vi "Datum draw.vi"(8 "error in (no error)":errorcluster, 10 "Details in":T1={"Angle"=0.0, "Reference"="", "Xoffset"=0, "Arc size"=0.0, "Measurment Name"="", "Pixel density"=0.0, "Circle"={"Point 1"={"X"=0.0, "Y"=0.0}, "Point 2"={"X"=0.0, "Y"=0.0}, "Center (Pixels)"={"X"=0.0, "Y"=0.0}, "Radius (Pixels)"=0.0}, "Color"=0, "Slanting line start"={"X"=0.0, "Y"=0.0}, "Sleeping line start"={"X"=0.0, "Y"=0.0}, "Mouse release"={"X"=0.0, "Y"=0.0}, "Line width"=0, "Small FOV?"=FALSE, "Fixed overlay details"={"Overlay coordinates"=[], "Config coordinates"=[], "Inspection mode?"=TRUE}, "PM angle"=0.0}, 11 "Image in":T2) -> (0 "error out":errorcluster, 1 "Overlay coordinates out":cluster{"X":dbl, "Y":dbl}[](array[cluster]), 2 "Text origin":cluster{"X":sgl, "Y":sgl}, 3 "Image out":T2)   [LabVIEW 2019]
uses:
  <vilib>/vision/Image Controls.llb/IMAQ Image.ctl
  Controls/DatumLine draw.ctl
  <vilib>/vision/NI_Vision_Development_Module.lvlib
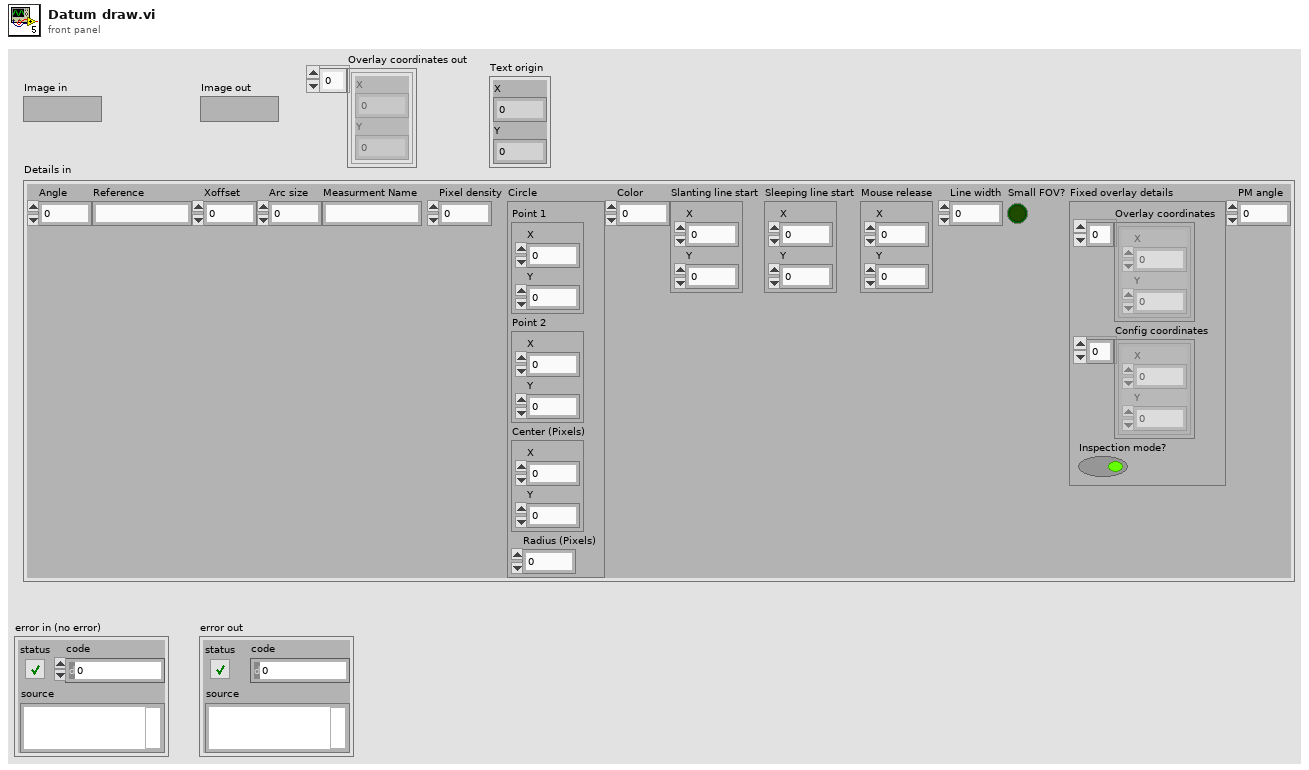
[diagram p1: front panel]
types:
  T1 = typedef "DatumLine draw.ctl" = cluster{"Angle":dbl, "Reference":string, "Xoffset":i32, "Arc size":dbl, "Measurment Name":string, "Pixel density":dbl, "Circle":cluster{"Point 1":cluster{"X":sgl, "Y":sgl}, "Point 2":cluster{"X":sgl, "Y":sgl}, "Center (Pixels)":cluster{"X":sgl, "Y":sgl}, "Radius (Pixels)":dbl}, "Color":u32, "Slanting line start":cluster{"X":sgl, "Y":sgl}, "Sleeping line start":cluster{"X":sgl, "Y":sgl}, "Mouse release":cluster{"X":sgl, "Y":sgl}, "Line width":i32, "Small FOV?":bool, "Fixed overlay details":cluster{"Overlay coordinates":cluster{"X":dbl, "Y":dbl}[], "Config coordinates":cluster{"X":dbl, "Y":dbl}[], "Inspection mode?":bool}, "PM angle":dbl}
  T2 = typedef "IMAQ Image.ctl" = refnum<image>
  T3 = cluster{"Overlay coordinates":cluster{"X":dbl, "Y":dbl}[], "Config coordinates":cluster{"X":dbl, "Y":dbl}[], "Inspection mode?":bool}
  T4 = cluster{"Center (Pixels)":cluster{"X":sgl, "Y":sgl}, "Radius (Pixels)":dbl}
  T5 = cluster{"Point 1":cluster{"X":sgl, "Y":sgl}, "Point 2":cluster{"X":sgl, "Y":sgl}, "Center (Pixels)":cluster{"X":sgl, "Y":sgl}, "Radius (Pixels)":dbl}
  T6 = cluster{"Desired Font (Application)":enum16{"User-specified Font", "Application Font", "System Font", "Dialog Font"}, "[User-specified Font]":cluster{"Font Name":string, "Size":i16, "Strikeout?":bool, "Italic?":bool, "Underline?":bool, "Outline?":bool, "Shadow?":bool, "Bold?":bool, "Rotation Angle":dbl}, "Horizontal Alignment":i16, "Vertical Alignment":i16}
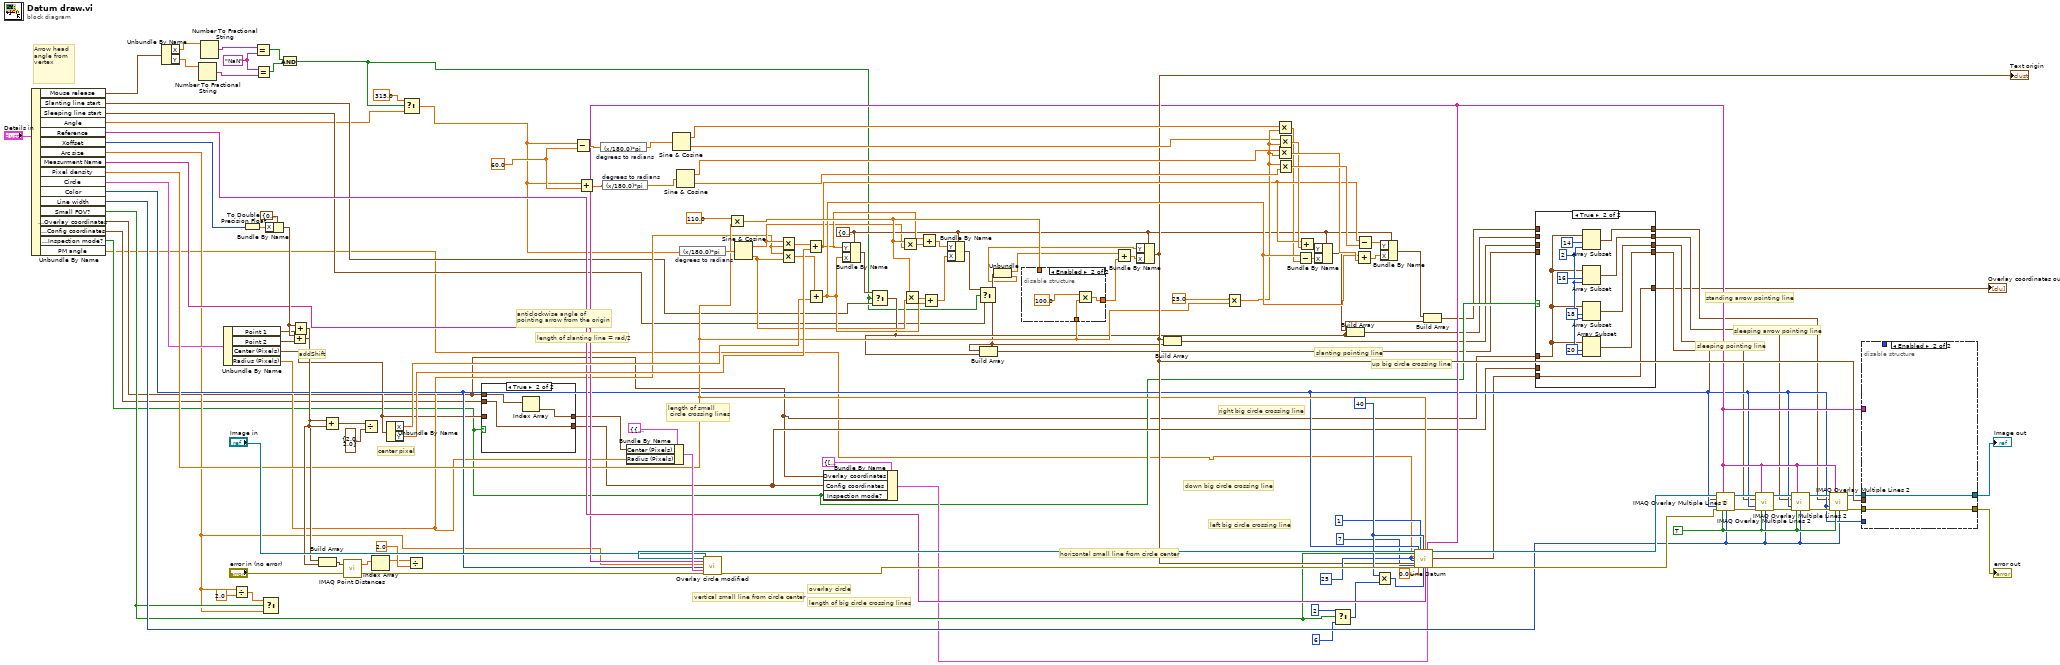
[diagram p0: block diagram]
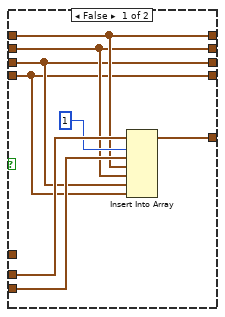
[diagram p2: hidden frame]
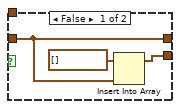
[diagram p3: hidden frame]
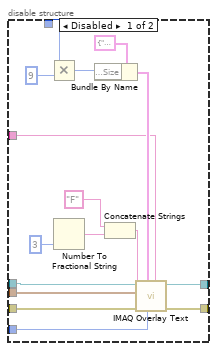
[diagram p4: hidden frame]
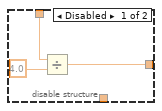
[diagram p5: hidden frame]
diagram:
  w44 = "NaN" ("x")
  w134 = TRUE ("Maintain Width?")
  w126 = u16 40 ("sleeping line length(in pixels)")
  w124 = u16 25 ("half Datum arrow width( in pixels)")
  w104 = 60.0
  w72 = cluster{"X":sgl, "Y":sgl} {"X"=0.0, "Y"=0.0} ("Point 1")
  # "Arrow head\nangle from vertex"
  # "length of slanting line = rad/2"
  # "length of small\n circle crossing lines"
  # "length of big circle crossing lines"
  # "anticlockwise angle of\npointing arrow from the origin"
  # "standing arrow pointing line"
  # "sleeping arrow pointing line"
  # "sleeping pointing line"
  # "slanting pointing line"
  # "vertical small line from circle center"
  # "horizontal small line from circle center"
  # "left big circle crossing line"
  # "right big circle crossing line"
  # "down big circle crossing line"
  # "up big circle crossing line"
  # "addShift"
  # "center pixel"
  # "overlay circle"
  n1 = Unbundle By Name("Details in") -> ("Mouse release"=w49:cluster{"X":sgl, "Y":sgl}, "Slanting line start"=w38:cluster{"X":sgl, "Y":sgl}, "Sleeping line start"=w37:cluster{"X":sgl, "Y":sgl}, "Angle"=w3:dbl, "Reference"=w56:string, "Xoffset"=w55:i32, "Arc size"=w24:dbl, "Measurment Name"=w54:string, "Pixel density"=w53:dbl, "Circle"=w52:T5, "Color"=w51:u32, "Line width"=w31:i32, "Small FOV?"=w27:bool, "Fixed overlay details.Overlay coordinates"=w5:cluster{"X":dbl, "Y":dbl}[], "Fixed overlay details.Config coordinates"=w20:cluster{"X":dbl, "Y":dbl}[], "Fixed overlay details.Inspection mode?"=w15:bool, "PM angle"=w1:dbl)
  n2 = Unbundle By Name(w49) -> ("X"=w48:sgl, "Y"=w47:sgl)
  n3 = Number To Fractional String(number=w47) -> (F-format string=w45:string)  [unwired: 3 in]
  n4 = Number To Fractional String(number=w48) -> (F-format string=w46:string)  [unwired: 3 in]
  n5 = Unbundle By Name(w52) -> ("Point 1"=w86:cluster{"X":sgl, "Y":sgl}, "Point 2"=w88:cluster{"X":sgl, "Y":sgl}, "Center (Pixels)"=w23:cluster{"X":sgl, "Y":sgl}, "Radius (Pixels)"=w50:dbl)
  n6 = Divide(x=w24, y=2.0) -> (x/y=w25:dbl)
  n7 = To Double Precision Float(number=w55) -> (double precision float=w85:dbl)
  n8 = Equal?(x=w46, y=w44) -> (x = y?=w43:bool)
  n9 = Equal?(x=w44, y=w45) -> (x = y?=w42:bool)
  n10 = Select(t=w25, s=w27, f=w24) -> ()  [unwired: 1 out]
  n11 = Bundle By Name(cluster=cluster{"X":sgl, "Y":sgl} {"X"=0.0, "Y"=0.0} ("Angle.Point 2a"), "X"=w85) -> (w87:cluster{"X":sgl, "Y":sgl})
  n12 = And(x=w43, y=w42) -> (x .and. y?=w36:bool)
  n13 = Add(x=w87, y=w88) -> (x+y=w92:cluster{"X":sgl, "Y":sgl})
  n14 = Add(x=w87, y=w86) -> (x+y=w91:cluster{"X":sgl, "Y":sgl})
  n15 = Build Array(w91, w92) -> (w93:cluster{"X":sgl, "Y":sgl}[])
  n16 = Add(x=w91, y=w92) -> (x+y=w89:cluster{"X":sgl, "Y":sgl})
  n17 = call "IMAQ Point Distances"("Points"=w93, "error in (no error)"="error in (no error)") -> ("Distances"=w94:sgl[], "error out"=w128:errorcluster)  [unwired: 3 in]
  n18 = Divide(x=w89, y=cluster{"X":sgl, "Y":sgl} {"X"=2.0, "Y"=2.0}) -> ()  [unwired: 1 out]
  n19 = Index Array(array=w94) -> (element=w95:sgl)  [unwired: 1 in]
  n20 = Unbundle By Name(w23) -> ("X"=w98:sgl, "Y"=w99:sgl)
  n21 = Select(t=315.0, s=w36, f=w3) -> (s? t:f=w2:dbl)
  n22 = Divide(x=w95, y=sgl 2.0) -> ()  [unwired: 1 out]
  n23 = case shown="True" w15 {
    tunnel: w23 -> [w135 _]
    tunnel: [w135 w139] -> w22
    tunnel: w5 -> [_ w140]
    tunnel: w20 -> [_ w138]
    tunnel: [w136 w138] -> w17
    frame False {
      n24 = Insert Into Array(array=cluster{"X":sgl, "Y":sgl}[] [], new element=w135) -> (w136:cluster{"X":sgl, "Y":sgl}[])  [unwired: 1 in]
    }
    frame True {
      n25 = Index Array(array=w140) -> (element=w139:cluster{"X":dbl, "Y":dbl})  [unwired: 1 in]
    }
  }
  n26 = Subtract(x=w2, y=w104) -> (x-y=w105:dbl)
  n27 = Add(x=w2, y=w104) -> (x+y=w106:dbl)
  n28 = expression code="(x/180.0)*pi" "degrees to radians"(w105) -> (w120:dbl)
  n29 = expression code="(x/180.0)*pi" "degrees to radians"(w106) -> (w121:dbl)
  n30 = Bundle By Name(cluster=T4 {"Center (Pixels)"={"X"=0.0, "Y"=0.0}, "Radius (Pixels)"=0.0} ("Circle center"), "Center (Pixels)"=w22, "Radius (Pixels)"=w50) -> (w133:T4)
  n31 = Sine & Cosine(0:w120) -> (1:w107:dbl, 2:w108:dbl)
  n32 = Sine & Cosine(0:w121) -> (1:w113:dbl, 2:w114:dbl)
  n33 = expression code="(x/180.0)*pi" "degrees to radians"(w2) -> (w58:dbl)
  n34 = call "Overlay circle modified.vi"("Image In"="Image in", "Measurment Name"=w54, "Overlay width"=w24, "Overlay color"=w51, "Circle center"=w133, "error in (no error)"=w128) -> ("Image out"=w131:T2, "error out"=w129:errorcluster)  [unwired: 12 in]
  n35 = Multiply(x=sgl 110.0, y=w53) -> (x*y=w123:dbl)
  n36 = Sine & Cosine(0:w58) -> (1:w59:dbl, 2:w60:dbl)
  n37 = Multiply(x=w59, y=w50) -> (x*y=w78:dbl)
  n38 = Multiply(x=w50, y=w60) -> (x*y=w79:dbl)
  n39 = Add(x=w78, y=w99) -> (x+y=w110:dbl)
  n40 = Add(x=w79, y=w98) -> (x+y=w115:dbl)
  n41 = Bundle By Name(cluster=T3 {"Overlay coordinates"=[], "Config coordinates"=[], "Inspection mode?"=TRUE} ("Fixed overlay details 2"), "Overlay coordinates"=w5, "Config coordinates"=w17, "Inspection mode?"=w15) -> (w19:T3)
  n42 = Bundle By Name(cluster=w72, "Y"=w110, "X"=w115) -> (w41:cluster{"X":sgl, "Y":sgl})
  n43 = Select(t=w41, s=w36, f=w38) -> (s? t:f=w40:cluster{"X":sgl, "Y":sgl})
  n44 = Multiply(x=w123, y=w59) -> (x*y=w61:dbl)
  n45 = Multiply(x=w123, y=w60) -> (x*y=w62:dbl)
  n46 = Add(x=w110, y=w61) -> (x+y=w68:dbl)
  n47 = Add(x=w62, y=w115) -> (x+y=w69:dbl)
  n48 = Bundle By Name(cluster=w72, "Y"=w68, "X"=w69) -> (w39:cluster{"X":sgl, "Y":sgl})
  n49 = Select(t=w39, s=w36, f=w37) -> (s? t:f=w34:cluster{"X":sgl, "Y":sgl})
  n50 = Build Array(w34, w40) -> (w8:cluster{"X":sgl, "Y":sgl}[])
  n51 = Unbundle(w34) -> ("X"=w33:sgl, "Y"=w32:sgl)
  n52 = disable-structure shown="Enabled" {
    disable-tunnel: [w142 w144] -> w65
    disable-tunnel: w123 -> [w141 _]
    disable-tunnel: w53 -> [_ w145]
    frame Disabled {
      n53 = Divide(x=w141, y=4.0) -> (x/y=w142:dbl)
    }
    frame Enabled {
      n54 = Multiply(x=100.0, y=w145) -> (x*y=w144:dbl)
    }
  }
  n55 = Add(x=w33, y=w65) -> (x+y=w66:dbl)
  n56 = Bundle By Name(cluster=w72, "Y"=w32, "X"=w66) -> (w100:cluster{"X":sgl, "Y":sgl})
  "Text origin" <- w100
  n57 = Build Array(w100, w34) -> (w10:cluster{"X":sgl, "Y":sgl}[])
  n58 = Multiply(x=sgl 25.0, y=w53) -> (x*y=w112:dbl)
  n59 = Multiply(x=w107, y=w112) -> (x*y=w109:dbl)
  n60 = Multiply(x=w113, y=w112) -> (x*y=w116:dbl)
  n61 = Multiply(x=w108, y=w112) -> (x*y=w111:dbl)
  n62 = Multiply(x=w112, y=w114) -> (x*y=w117:dbl)
  n63 = Subtract(x=w115, y=w109) -> (x-y=w67:dbl)
  n64 = Add(x=w110, y=w111) -> (x+y=w118:dbl)
  n65 = Bundle By Name(cluster=w72, "Y"=w118, "X"=w67) -> (w70:cluster{"X":sgl, "Y":sgl})
  n66 = Select(t=u16 2 ("y"), s=w27, f=u16 6 ("y")) -> (s? t:f=w28:u16)
  n67 = Build Array(w70, w40) -> (w12:cluster{"X":sgl, "Y":sgl}[])
  n68 = Add(x=w115, y=w116) -> (x+y=w119:dbl)
  n69 = Subtract(x=w110, y=w117) -> (x-y=w71:dbl)
  n70 = Multiply(x=w126, y=w28) -> (x*y=w127:u16)
  n71 = Bundle By Name(cluster=w72, "Y"=w71, "X"=w119) -> (w73:cluster{"X":sgl, "Y":sgl})
  n72 = call "Line Datum.vi"("Image in"=w131, "Small FOV?"=w27, "Angle of rotation"=w1, "half Datum arrow width( in pixels)"=w124, "Arrow height (in pixels)"=w124, "Datum origin"=w100, "Start index"=7, "error in (no error)"=w129, "Color"=w51, "Datum line angle"=0.0, "Box start index"=1, "sleeping line length(in pixels)"=w126, "Angular line length(in pixels)"=w127, "pixel factor"=w53, "Reference string"=w56, "Measurement name"=w54, "Fixed overlay details"=w19) -> ("Image out"=w102:T2, "Overlay coordinates out"=w16:cluster{"X":dbl, "Y":dbl}[], "error out"=w101:errorcluster)  [unwired: 7 in, 1 out]
  n73 = Build Array(w73, w40) -> (w14:cluster{"X":sgl, "Y":sgl}[])
  n74 = case shown="True" w15 {
    tunnel: w14 -> [w150 _]
    tunnel: w12 -> [w149 _]
    tunnel: w10 -> [w148 _]
    tunnel: w8 -> [w147 _]
    tunnel: w17 -> [w154 _]
    tunnel: w16 -> [w153 w165]
    tunnel: [w151 w165] -> w6
    tunnel: [w150 w159] -> w13
    tunnel: [w149 w158] -> w11
    tunnel: [w148 w157] -> w9
    tunnel: [w147 w156] -> w7
    tunnel: w5 -> [_ w155]
    frame False {
      n75 = Insert Into Array(array=w154, index=1, new element #1=w153, new element #2=w150, new element #3=w149, new element #4=w148, new element #5=w147) -> (w151:cluster{"X":dbl, "Y":dbl}[])
    }
    frame True {
      w162 = 2 ("length")
      n76 = Array Subset(array=w155, index=14, length=w162) -> (w159:cluster{"X":dbl, "Y":dbl}[])
      n77 = Array Subset(array=w155, index=16, length=w162) -> (w158:cluster{"X":dbl, "Y":dbl}[])
      n78 = Array Subset(array=w155, index=18, length=w162) -> (w157:cluster{"X":dbl, "Y":dbl}[])
      n79 = Array Subset(array=w155, index=20, length=w162) -> (w156:cluster{"X":dbl, "Y":dbl}[])
    }
  }
  "Overlay coordinates out" <- w6
  n80 = call "IMAQ Overlay Multiple Lines 2"("Image"=w102, "Group"=w54, "Line End Points"=w7, "Color"=w51, "error in (no error)"=w101, "Maintain Width?"=w134, "Width"=w31) -> ("Image Out"=w64:T2, "error out"=w63:errorcluster)  [unwired: 7 in]
  n81 = call "IMAQ Overlay Multiple Lines 2"("Image"=w64, "Group"=w54, "Line End Points"=w9, "Color"=w51, "error in (no error)"=w63, "Maintain Width?"=w134, "Width"=w31) -> ("Image Out"=w75:T2, "error out"=w74:errorcluster)  [unwired: 7 in]
  n82 = call "IMAQ Overlay Multiple Lines 2"("Image"=w75, "Group"=w54, "Line End Points"=w11, "Color"=w51, "error in (no error)"=w74, "Maintain Width?"=w134, "Width"=w31) -> ("Image Out"=w76:T2, "error out"=w77:errorcluster)  [unwired: 7 in]
  n83 = call "IMAQ Overlay Multiple Lines 2"("Image"=w76, "Group"=w54, "Line End Points"=w13, "Color"=w51, "error in (no error)"=w77, "Maintain Width?"=w134, "Width"=w31) -> ("Image Out"=w82:T2, "error out"=w80:errorcluster)  [unwired: 7 in]
  n84 = disable-structure shown="Enabled" {
    disable-tunnel: w80 -> [w182 w184]
    disable-tunnel: [w181 w184] -> w81
    disable-tunnel: w82 -> [w180 w183]
    disable-tunnel: [w179 w183] -> w83
    disable-tunnel: w54 -> [w169 _]
    disable-tunnel: w100 -> [w168 _]
    disable-tunnel: w51 -> [w167 _]
    disable-tunnel: _ -> [w166 _]
    frame Disabled {
      n85 = Multiply(x=w166, y=u8 9) -> (x*y=w170:u8)
      n86 = Number To Fractional String(precision (6)=i16 3) -> (number=w174:dbl, F-format string=w175:string)  [unwired: 2 in]
      n87 = Bundle By Name(cluster=T6 {"Desired Font (Application)"=enum."User-specified Font", "[User-specified Font]"={"Font Name"="Symbol", "Size"=130, "Strikeout?"=FALSE, "Italic?"=FALSE, "Underline?"=FALSE, "Outline?"=FALSE, "Shadow?"=FALSE, "Bold?"=TRUE, "Rotation Angle"=0.0}, "Horizontal Alignment"=0, "Vertical Alignment"=2} ("Font, Size & Style"), "[User-specified Font].Size"=w170) -> (w172:T6)
      n88 = Concatenate Strings("F" ("string"), w175) -> (w177:string)
      n89 = call "IMAQ Overlay Text"("Group"=w169, "Text Color (black)"=w167, "Font, Size & Style"=w172, "error in (no error)"=w182, "String"=w177, "Origin"=w168, "Image"=w180) -> ("error out"=w181:errorcluster, "Image Out"=w179:T2)  [unwired: 3 in]
    }
    frame Enabled {
    }
  }
  "Image out" <- w83
  "error out" <- w81
